vi "1D array remove NaN.vi"(1 "Array input":dbl[](array[numeric])=[nan, 2.0, nan, 4.0, 5.0, nan, nan] format="%.2e", 2 "delete Nan":bool) -> (0 "cleaned array":dbl[](array[numeric])=[2.0, 2.0, 2.0, 4.0, 5.0, 5.0, 5.0])   [LabVIEW 2020]
panel:
  # "Inspect the array and either \n(1) replace a NaN with the nearest non-NaN value in the array. \nor (2) delete the NaN\n\nNote) A single NaN in the array can make lots of built-in mathematics VI's unreliable or useless."
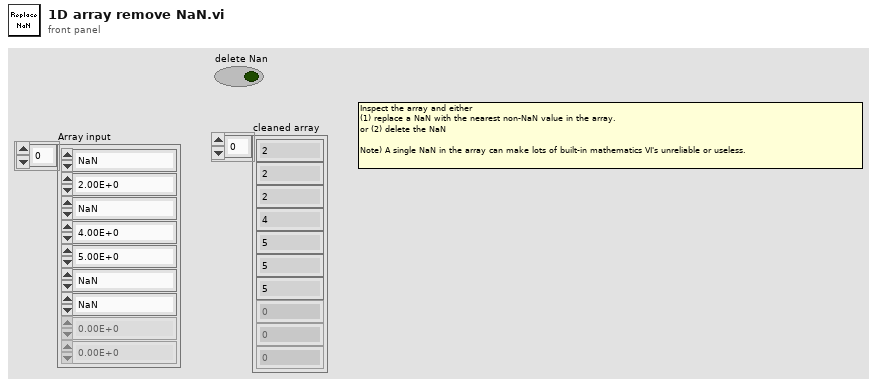
[diagram p1: front panel]
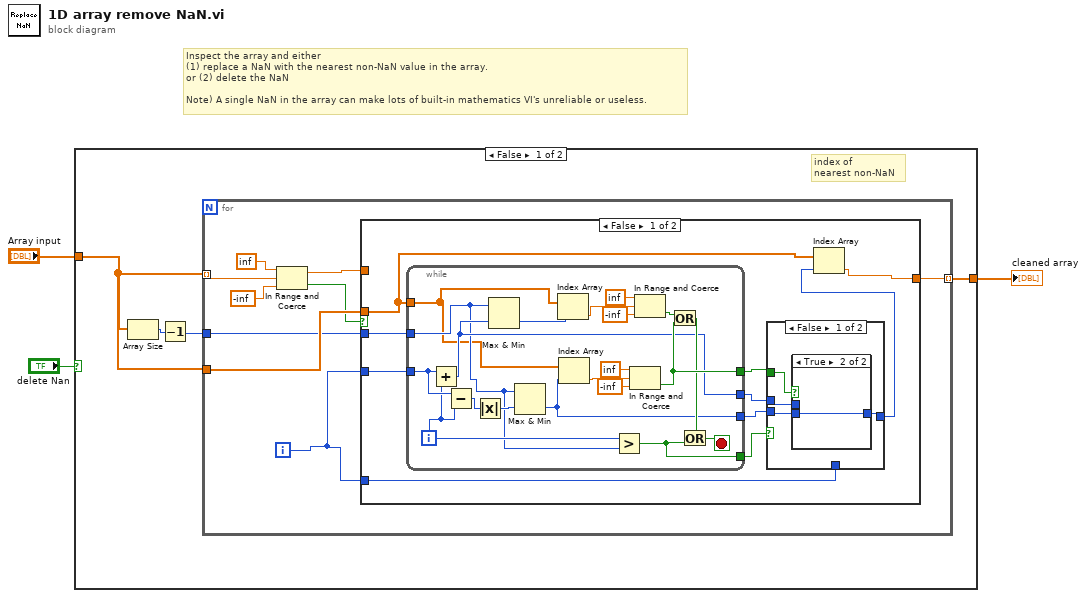
[diagram p0: block diagram]
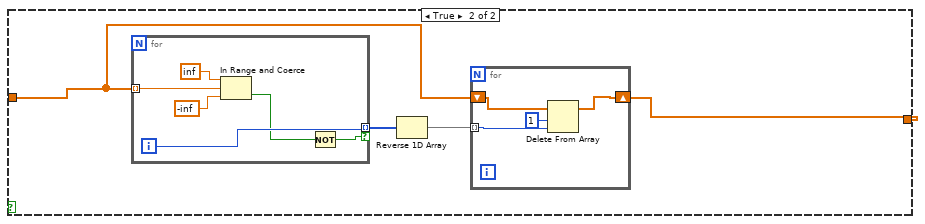
[diagram p5: hidden frame]
diagram:
  # "Inspect the array and either \n(1) replace a NaN with the nearest non-NaN value in the array. \nor (2) delete the NaN\n\nNote) A single NaN in the array can make lots of built-in mathematics VI's unreliable or useless."
  n1 = case shown="False" "delete Nan" {
    tunnel: [w7 w56] -> w3
    tunnel: "Array input" -> [w6 w57]
    frame False {
      # "index of\nnearest non-NaN"
      n2 = Array Size(array=w6) -> (size(s)=w5:i32)
      n3 = Decrement(x=w5) -> (x-1=w4:i32)
      n4 = for {
        tunnel: w6 -> [w14] mode=indexing
        tunnel: w6 -> [w13]
        tunnel: [w11] -> w7 mode=indexing
        tunnel: w4 -> [w8]
        i -> [w9]
        n5 = In Range and Coerce(upper limit=inf, x=w14, lower limit=-inf) -> (coerced(x)=w10:dbl, In Range?=w12:bool)
        n6 = case shown="False" w12 {
          tunnel: w13 -> [w25 _]
          tunnel: [w22 w54] -> w11
          tunnel: w10 -> [_ w54]
          tunnel: w9 -> [w26 _]
          tunnel: w9 -> [w19 _]
          tunnel: w8 -> [w17 _]
          frame False {
            n7 = while {
              tunnel: w25 -> [w34]
              tunnel: w26 -> [w50]
              tunnel: [w45] -> w18
              tunnel: [w36] -> w23
              tunnel: [w40] -> w21
              tunnel: [w41] -> w20
              tunnel: w17 -> [w35]
              i -> [w44]
              stop <- w42 stop-if-true
              n8 = Add(x=w50, y=w44) -> (x+y=w40:i32)
              n9 = Subtract(x=w50, y=w44) -> (x-y=w39:i32)
              n10 = Absolute Value(x=w39) -> (abs(x)=w37:i32)
              n11 = Max & Min(x=w35, y=w40) -> (min(x,y)=w38:i32)  [unwired: 1 out]
              n12 = Max & Min(x=w35, y=w37) -> (min(x,y)=w36:i32)  [unwired: 1 out]
              n13 = Index Array(array=w34, index=w38) -> (element=w51:dbl)
              n14 = Index Array(array=w34, index=w36) -> (element=w47:dbl)
              n15 = Greater?(x=w44, y=w35) -> (0:w41:bool)
              n16 = In Range and Coerce(upper limit=inf, x=w47, lower limit=-inf) -> (In Range?=w45:bool)  [unwired: 1 out]
              n17 = In Range and Coerce(upper limit=inf, x=w51, lower limit=-inf) -> (In Range?=w46:bool)  [unwired: 1 out]
              n18 = Or(x=w46, y=w45) -> (x .or. y?=w43:bool)
              n19 = Or(x=w43, y=w41) -> (x .or. y?=w42:bool)
            }
            n20 = case shown="False" w20 {
              tunnel: [w30 w33] -> w24
              tunnel: w23 -> [w29 _]
              tunnel: w21 -> [w28 _]
              tunnel: w19 -> [_ w33]
              tunnel: w18 -> [w27 _]
              frame False {
                n21 = case shown="True" w27 {
                  tunnel: [w31 w32] -> w30
                  tunnel: w29 -> [_ w32]
                  tunnel: w28 -> [w31 _]
                  frame False {
                  }
                  frame True {
                  }
                }
              }
              frame True {
              }
            }
            n22 = Index Array(array=w25, index=w24) -> (element=w22:dbl)
          }
          frame True {
          }
        }
      }
    }
    frame True {
      n23 = for {
        tunnel: w57 -> [w66] mode=indexing
        tunnel: [w65] -> w58 mode=indexing if=w63
        i -> [w65]
        n24 = In Range and Coerce(upper limit=inf, x=w66, lower limit=-inf) -> (In Range?=w64:bool)  [unwired: 1 out]
        n25 = Not(x=w64) -> (.not. x?=w63:bool)
      }
      n26 = Reverse 1D Array(array=w58) -> (reversed array=w55:i32[])
      n27 = for {
        tunnel: w55 -> [w59] mode=indexing
        shift-right: [w61] -> w56
        shift-left: w57 -> [w62]
        n28 = Delete From Array(array=w62, length=1, index=w59) -> (array with subset deleted=w61:dbl[])  [unwired: 1 out]
      }
    }
  }
  "cleaned array" <- w3
